vi "Instrumento_caracterizacion.vi"() -> ()   [LabVIEW 2009]
uses:
  <vilib>/picture/picture.llb/imagedata.ctl
  <vilib>/Analysis/NI_AALBase.lvlib
panel:
  out "CamControl":refnum<k7>
  in  "Configurar para franjas":bool
  in  "Load properties":bool
  in  "Save properties":bool
  in  "VCD Properties":bool
  in  "Directorio scripts matlab":path=path "C:/Users/franjas/Documents/rutinas-calibracion-slm"
  in  "File to load":path
  in  "File to save":path
  in  "Exit":bool
  out "Exit live 2":bool
  out "Live Picture 2":picture
  out "image data":T1
  out "Histogram Graph":T2(graph)
  out "Current exposure value":i32
  in  "Run live preview":bool
  out "Exit live":bool
  out "Live Picture":picture
  out "Video formats":string[](array[string])
  out "Devices":string[](array[string])
  in  "ICImagingControl":refnum<k7>(container)
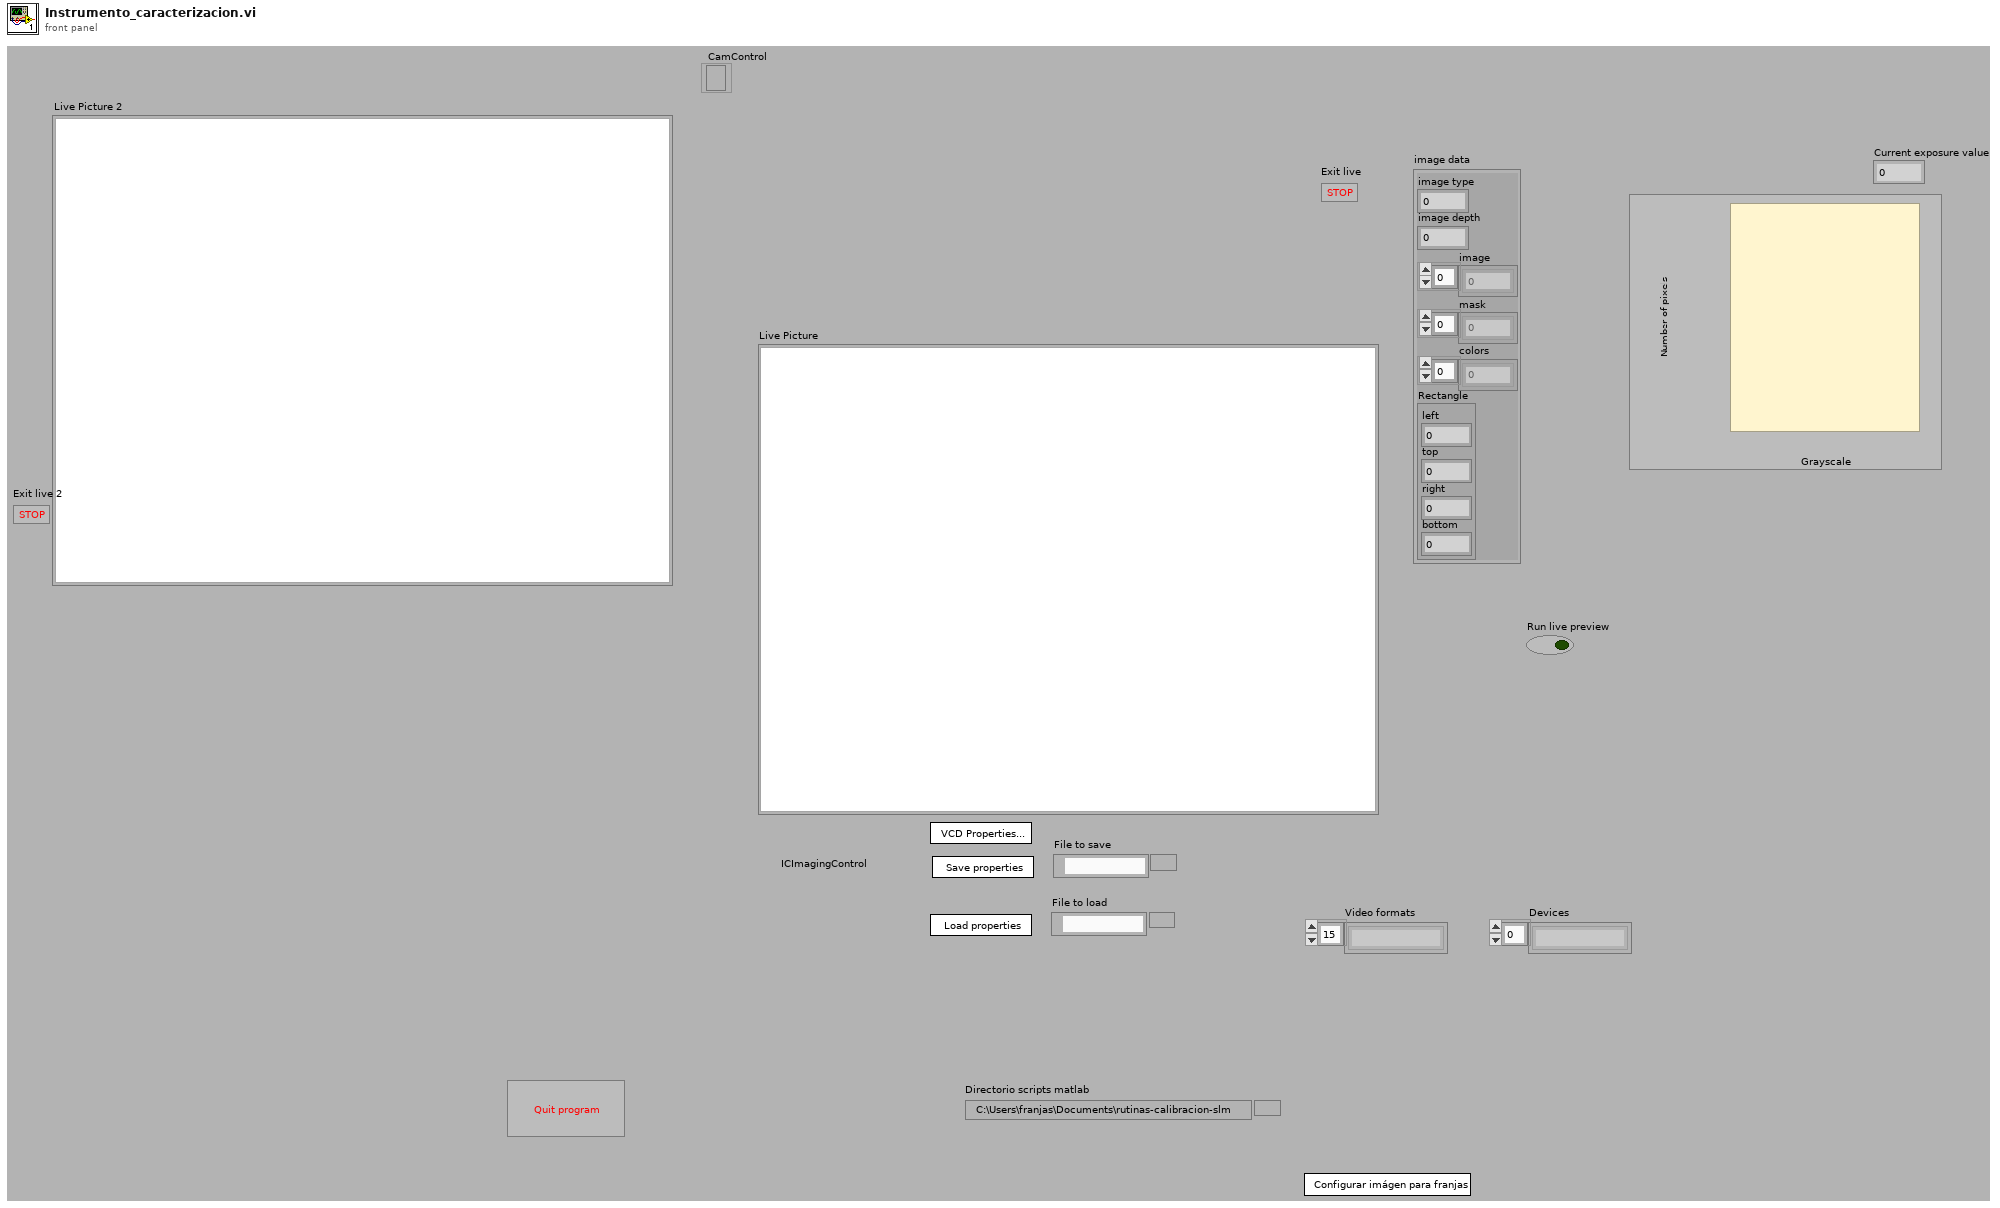
[diagram p1: front panel]
types:
  T1 = typedef "imagedata.ctl" = cluster{"image type":i32, "image depth":i32, "image":u8[], "mask":u8[], "colors":u32[], "Rectangle":cluster{"left":i16, "top":i16, "right":i16, "bottom":i16}}
  T2 = cluster{"X Values":dbl[], "Histogram: h(x)":i32[]}
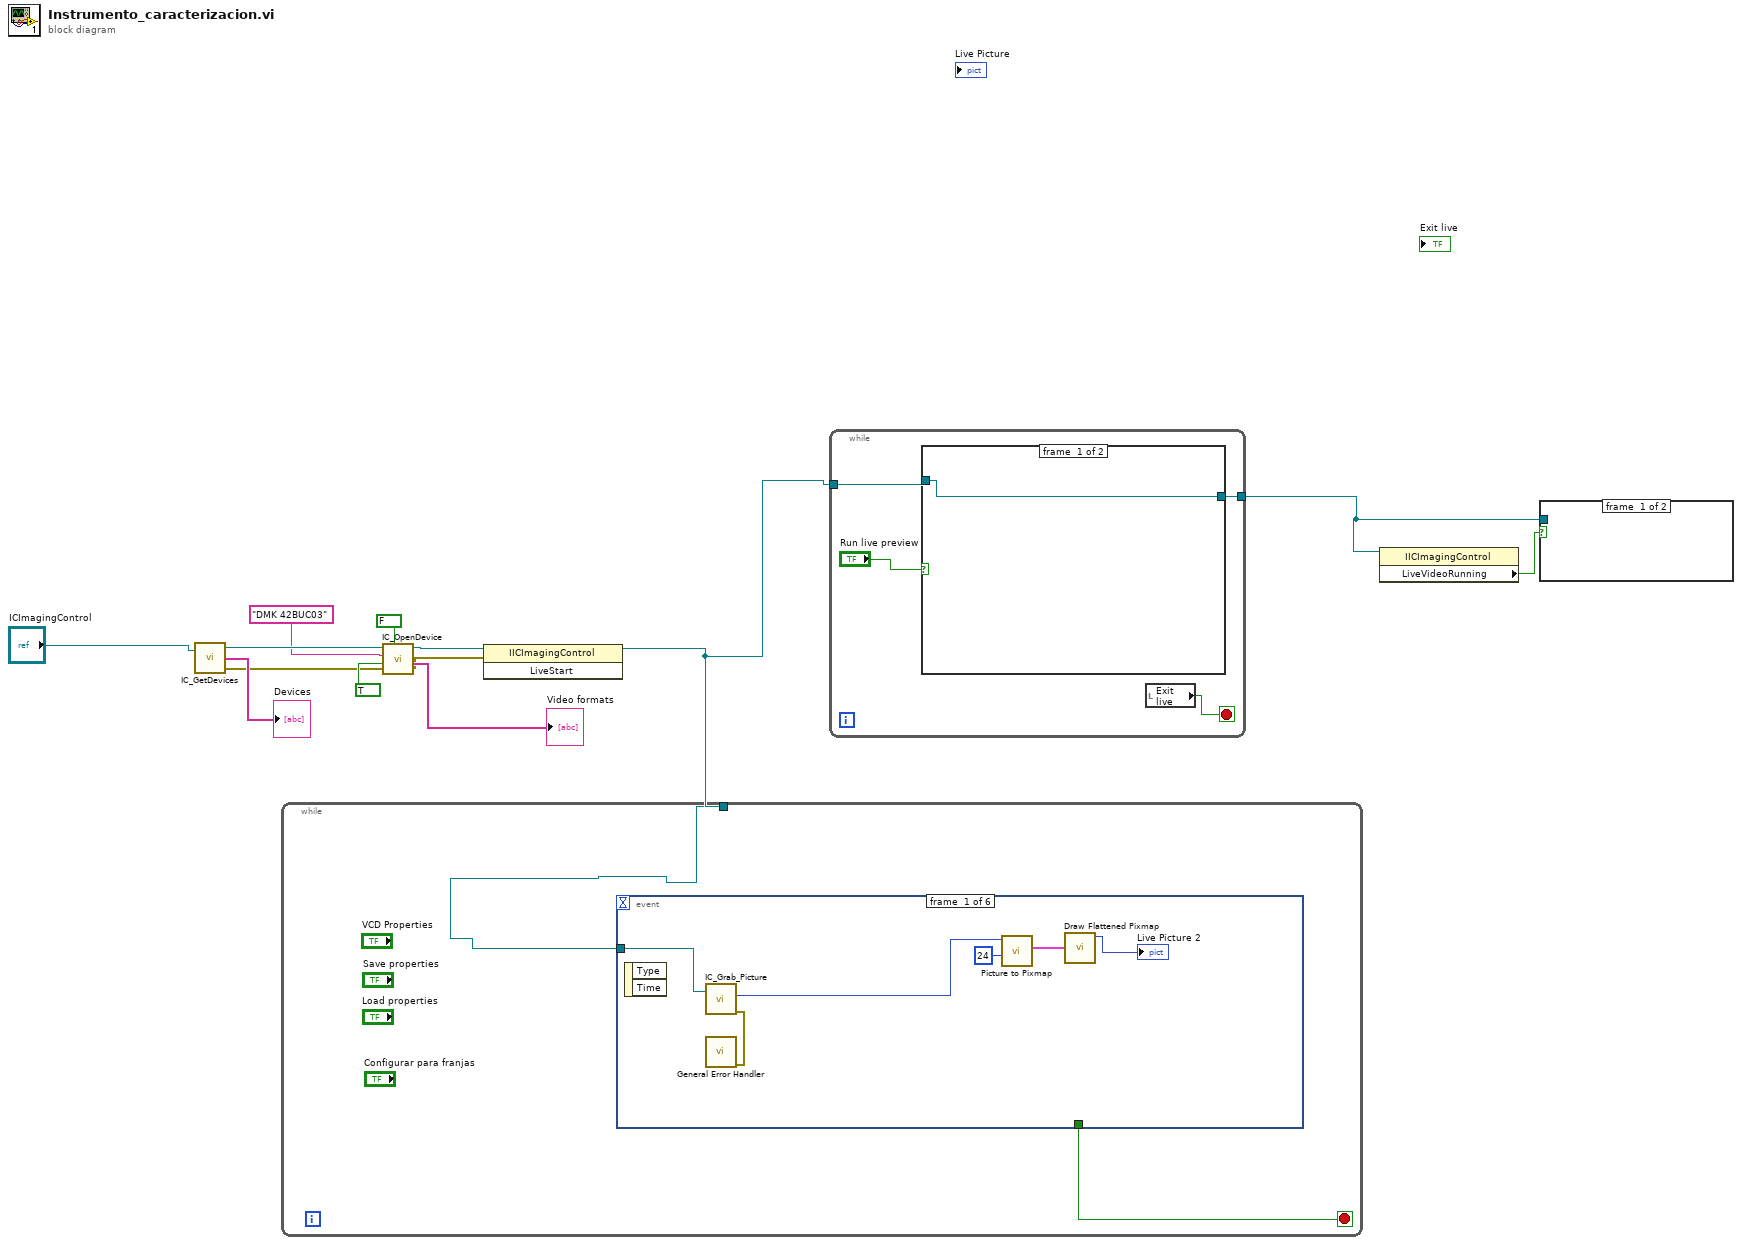
[diagram p0: block diagram]
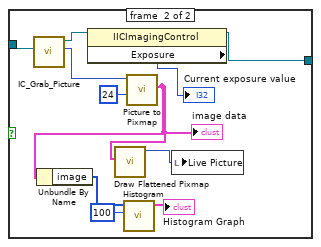
[diagram p2: hidden frame]
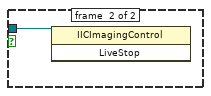
[diagram p3: hidden frame]
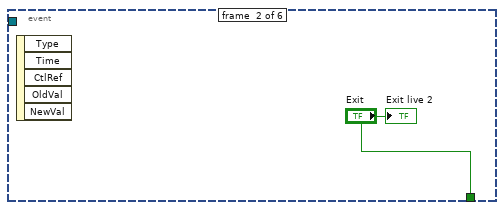
[diagram p4: hidden frame]
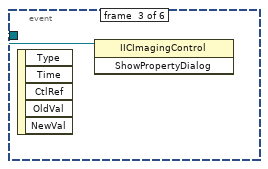
[diagram p5: hidden frame]
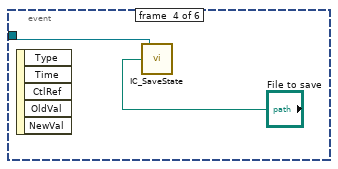
[diagram p6: hidden frame]
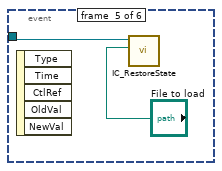
[diagram p7: hidden frame]
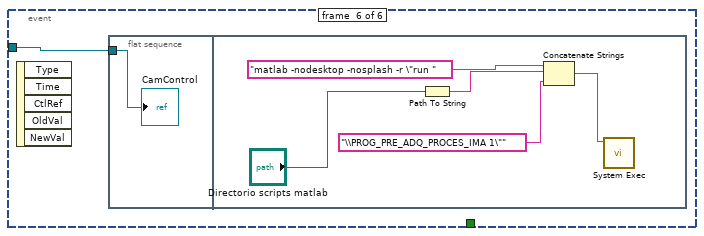
[diagram p8: hidden frame]
diagram:
  n1 = call <userlib>:"IC_GetDevices.vi"("ICImagingControl In"="ICImagingControl") -> ("ICImagingControl Out"=w11:refnum<k7>, "Devices"=→"Devices":string[], "Error Out"=w2:errorcluster)  [unwired: 1 in]
  n2 = call <userlib>:"IC_OpenDevice.vi"("Color"=FALSE, "Error In (no error)"=w2, "Live"=TRUE, "Device"="DMK 42BUC03", "ICImagingControl In"=w11) -> ("VideoFormats"=→"Video formats":string[], "ICImagingControl Out"=w6:refnum<k7>, "Error Out"=w1:errorcluster)  [unwired: 1 in, 3 out]
  n3 = invoke class="IICImagingControl" method="LiveStart"(reference=w6, error in=w1) -> (reference out=w3:refnum<k7>)  [unwired: 1 in, 2 out]
  n4 = while {
    tunnel: w3 -> [w15]
    stop <- w14 stop-if-true
    n5 = event shown="[5] \"Configurar para franjas\": Value Change" {
      selector: _ -> [_ _ _ _ _ _]
      dyn-events: _ -> [_ _ _ _ _ _]
      timeout: _ -> [_ _ _ _ _ _]
      tunnel: w15 -> [w16 _ w23 w25 w27 w28]
      tunnel: [_ "Exit" _ _ _ _] -> w14
      event #0 {
        n6 = event-data() -> ()  [unwired: 1 in, 2 out]
        n7 = call <userlib>:"IC_Grab_Picture.vi"("ICImagingControl In"=w16) -> ("Picture Out"=w20:picture, "Error Out"=w21:errorcluster)  [unwired: 1 in, 2 out]
        n8 = call <vilib>:"General Error Handler.vi"("error in (no error)"=w21) -> ()  [unwired: 10 in, 5 out]
        n9 = call <vilib>:"Picture to Pixmap.vi"("depth"=24, "picture"=w20) -> ("image data"=w17:T1)  [unwired: 8 in, 1 out]
        n10 = call <vilib>:"Draw Flattened Pixmap.vi"("image data"=w17) -> ("new picture"=→"Live Picture 2":picture)  [unwired: 8 in]
      }
      event #1 {
        n11 = event-data() -> ()  [unwired: 1 in, 5 out]
        "Exit live 2" <- "Exit"
      }
      event #2 {
        n12 = event-data() -> ()  [unwired: 1 in, 5 out]
        n13 = invoke class="IICImagingControl" method="ShowPropertyDialog"(reference=w23) -> ()  [unwired: 2 in, 3 out]
      }
      event #3 {
        n14 = event-data() -> ()  [unwired: 1 in, 5 out]
        n15 = call <userlib>:"IC_SaveState.vi"("file path"="File to save", "ICImagingControl In"=w25) -> ()  [unwired: 1 in, 2 out]
      }
      event #4 {
        n16 = event-data() -> ()  [unwired: 1 in, 5 out]
        n17 = call <userlib>:"IC_RestoreState.vi"("File Path"="File to load", "ICImagingControl"=w27) -> ()  [unwired: 2 in, 2 out]
      }
      event #5 {
        n18 = event-data() -> ()  [unwired: 1 in, 5 out]
        n19 = flat-sequence {
          tunnel: w28 -> [w29]
          frame #0 {
            "CamControl" <- w29
          }
          frame #1 {
            n20 = Path To String(path="Directorio scripts matlab") -> (string=w34:string)
            n21 = Concatenate Strings("matlab -nodesktop -nosplash -r \"run " ("command line"), w34, "\\PROG_PRE_ADQ_PROCES_IMA 1\"" ("command line")) -> (w32:string)
            n22 = call <vilib>:"System Exec.vi"("command line"=w32) -> ()  [unwired: 7 in, 4 out]
          }
        }
      }
    }
  }
  n23 = while {
    tunnel: w3 -> [w37]
    tunnel: [w36] -> w4
    stop <- w38 stop-if-true
    n24 = case shown="True" "Run live preview" {
      tunnel: w37 -> [w39 w47]
      tunnel: [w39 w41] -> w36
      frame #0 {
      }
      frame #1 {
        n25 = call <userlib>:"IC_Grab_Picture.vi"("ICImagingControl In"=w47) -> ("ICImagingControl Out"=w42:refnum<k7>, "Picture Out"=w50:picture)  [unwired: 1 in, 2 out]
        n26 = property class="IICImagingControl"(reference=w42) -> (reference out=w41:refnum<k7>, "Exposure"=→"Current exposure value":i32)  [unwired: 1 in, 1 out]
        n27 = call <vilib>:"Picture to Pixmap.vi"("depth"=24, "picture"=w50) -> ("image data"=w46:T1)  [unwired: 8 in, 1 out]
        "image data" <- w46
        n28 = Unbundle By Name(w46) -> ("image"=w45:u8[])
        n29 = call <vilib>:"Draw Flattened Pixmap.vi"("image data"=w46) -> ("new picture"=w48:picture)  [unwired: 8 in]
        n30 = call <vilib>:"Histogram.vi"("intervals"=100, "X"=w45) -> ("Histogram Graph"=→"Histogram Graph":T2)  [unwired: 6 in, 3 out]
        n31 = local write "Live Picture"(w48) -> ()
      }
    }
    n32 = local read "Exit live"() -> (w38:bool)
  }
  n33 = property class="IICImagingControl"(reference=w4) -> ("LiveVideoRunning"=w5:bool)  [unwired: 1 in, 2 out]
  n34 = case shown="True" w5 {
    tunnel: w4 -> [_ w51]
    frame #0 {
    }
    frame #1 {
      n35 = invoke class="IICImagingControl" method="LiveStop"(reference=w51) -> ()  [unwired: 2 in, 3 out]
    }
  }
